vi "ACQ_TIMING_MODE - Type.vi"(8 "error in (no error)":errorcluster) -> (0 "error out":errorcluster, 3 "ACQ_TIMING_MODE_VALUE":i32)   [LabVIEW 2013]
doc: "<b>Buffer policy settings can be only unsafe in xiAPI LabVIEW library</b>\nUNSAFE : User gets pointer to internally allocated circle buffer and data may be overwritten by device.\nSAFE : Data from device will be copied to user allocated buffer or xiApi allocated memory."
uses:
  ACQ_TIMING_MODE.ctl
  C:/Projects/Cameras3.x/xiLib/xiLIB_64bit/xiLIB/xiCamLib/API/x64/xiApi.NETX64.dll
  xiLIB_64bit/xiLIB/xiCamLib/API/x64/xiApi.NETX64.dll
panel:
  in  "ACQ TIMING MODE":T1
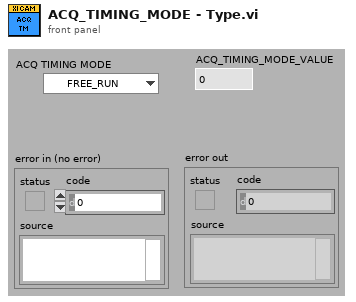
[diagram p1: front panel]
types:
  T1 = typedef "ACQ_TIMING_MODE.ctl" = enum16{"FREE_RUN", "FRAME_RATE"}
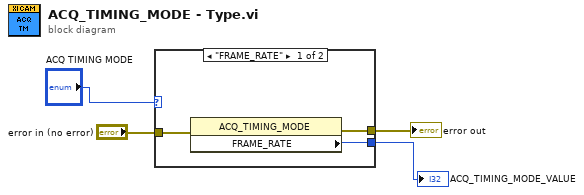
[diagram p0: block diagram]
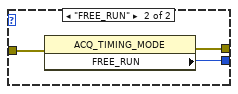
[diagram p2: hidden frame]
diagram:
  n1 = case shown="\"FRAME_RATE\"" "ACQ TIMING MODE" {
    tunnel: "error in (no error)" -> [w7 w10]
    tunnel: [w6 w9] -> w3
    tunnel: [w5 w8] -> w2
    frame "FRAME_RATE" {
      n2 = property class="ACQ_TIMING_MODE"(error in=w7) -> (error out=w6:errorcluster, "FRAME_RATE"=w5:i32)  [unwired: 1 in, 1 out]
    }
    frame "FREE_RUN" {
      n3 = property class="ACQ_TIMING_MODE"(error in=w10) -> (error out=w9:errorcluster, "FREE_RUN"=w8:i32)  [unwired: 1 in, 1 out]
    }
  }
  "error out" <- w3
  "ACQ_TIMING_MODE_VALUE" <- w2
